vi "convert h5 to csv.vi"(9 "delimiter":i8, 10 "csvfile":string, 11 "h5file":string) -> (1 "function return":i32, 2 "csvfile out":string, 3 "h5file out":string)   [LabVIEW 2019, in "apdm.lvlib"]
doc: "APDM_EXPORT int apdm_convert_h5_to_csv(char *h5file, char *csvfile, char delimiter);"
uses:
  apdm.lvlib
  Lee Lab/CP FES Walking 2018/Code/Working/LabVIEW/apdm.dll
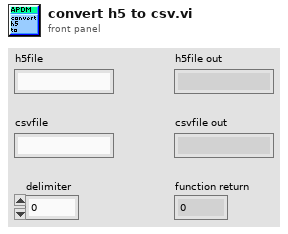
[diagram p1: front panel]
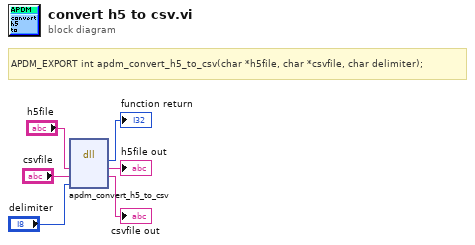
[diagram p0: block diagram]
diagram:
  # "APDM_EXPORT int apdm_convert_h5_to_csv(char *h5file, char *csvfile, char delimiter);"
  n1 = dll-call lib="C:/Users/jfalesi/Dropbox/Lee Lab/CP FES Walking 2018/Code/Working/LabVIEW/apdm.*" fn="apdm_convert_h5_to_csv"("h5file"="h5file", "csvfile"="csvfile", "delimiter"="delimiter") -> (→"function return":i32, "h5file"=→"h5file out":string, "csvfile"=→"csvfile out":string)  [unwired: 4 in, 2 out]
